vi "exercise8_writetoAO.vi"() -> ()   [LabVIEW 2018]
uses:
  <vilib>/DAQmx/write.llb/DAQmx Write (Analog DBL 1Chan 1Samp).vi
  <vilib>/DAQmx/create/channels.llb/DAQmx Create Channel (AO-Voltage-Basic).vi
  <vilib>/DAQmx/miscellaneous.llb/DAQmx Fill In Error Info.vi
panel:
  out "sampling rate":dbl
  out "error out":errorcluster
  in  "dt (ms)":u32=1
  in  "frequency (Hz)":dbl=1.0
  in  "physical channels":tag="Dev1/ao0"
  out "Waveform Graph":waveform(dbl)(graph)
  out "Waveform Chart":dbl(graph)
  in  "stop":bool
  # "SIGNAL GENERATION: WRITE TO ANALOG OUTPUT"
  # "CHANNEL"
  # "SIGNAL"
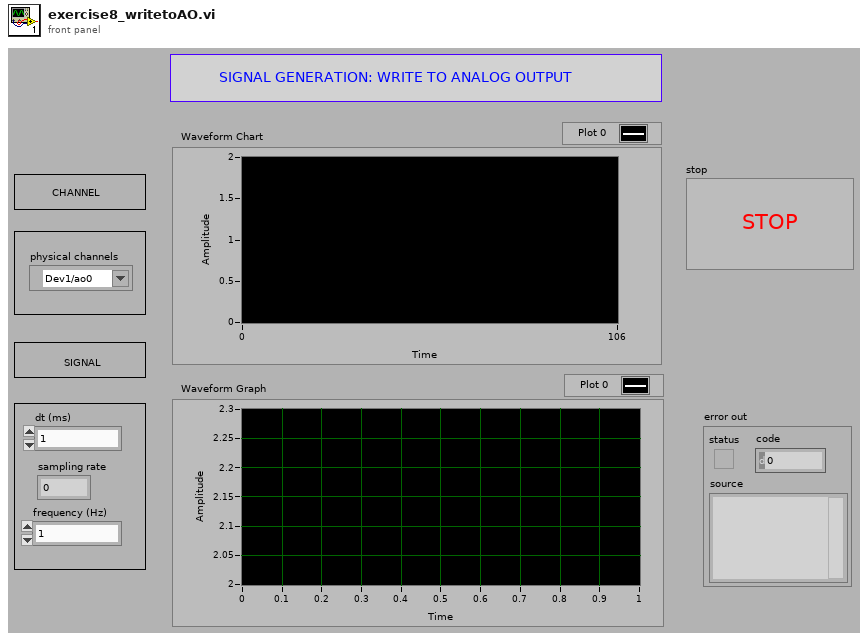
[diagram p1: front panel]
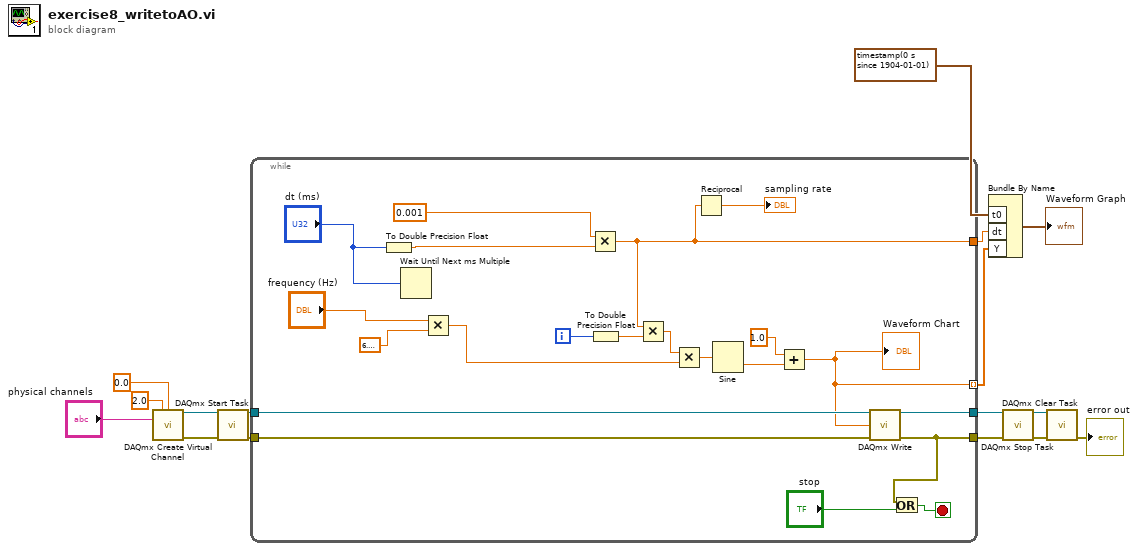
[diagram p0: block diagram]
diagram:
  n1 = call-poly <vilib>:"DAQmx Create Virtual Channel.vi"("maximum value"=2.0, "minimum value"=0.0, "physical channels"="physical channels") -> ("task out"=w9:refnum<k21>, "error out"=w8:errorcluster)  [unwired: 11 in]
  n2 = call <vilib>:"DAQmx Start Task.vi"("task/channels in"=w9, "error in"=w8) -> ("task out"=w16:refnum<k21>, "error out"=w15:errorcluster)  [unwired: 12 in]
  n3 = while {
    tunnel: w16 -> [w36]
    tunnel: w15 -> [w35]
    tunnel: [w37] -> w12
    tunnel: [w25] -> w11
    tunnel: [w33] -> w6 mode=indexing
    tunnel: [w22] -> w1
    i -> [w32]
    stop <- w27 stop-if-true
    n4 = To Double Precision Float(number="dt (ms)") -> (double precision float=w24:dbl)
    n5 = Wait Until Next ms Multiple(millisecond multiple="dt (ms)") -> ()  [unwired: 1 out]
    n6 = Multiply(x="frequency (Hz)", y=6.283185307179586) -> (x*y=w17:dbl)
    n7 = Multiply(x=0.001, y=w24) -> (x*y=w22:dbl)
    n8 = To Double Precision Float(number=w32) -> (double precision float=w30:dbl)
    n9 = Multiply(x=w22, y=w30) -> (x*y=w29:dbl)
    n10 = Multiply(x=w29, y=w17) -> (x*y=w28:dbl)
    n11 = Reciprocal(x=w22) -> (1/x=→"sampling rate":dbl)
    n12 = Sine(x=w28) -> (sin(x)=w34:dbl)
    n13 = Add(x=1.0, y=w34) -> (x+y=w33:dbl)
    "Waveform Chart" <- w33
    n14 = call-poly <vilib>:"DAQmx Write.vi"("task/channels in"=w36, "data"=w33, "error in"=w35) -> ("task out"=w37:refnum<k21>, "error out"=w25:errorcluster)  [unwired: 10 in, 1 out]
    n15 = Or(x=w25, y="stop") -> (x .or. y?=w27:bool)
  }
  n16 = Bundle By Name("t0"=timestamp(0 s since 1904-01-01), "dt"=w1, "Y"=w6) -> (→"Waveform Graph":waveform(dbl))  [unwired: 1 in]
  n17 = call <vilib>:"DAQmx Stop Task.vi"("task/channels in"=w12, "error in"=w11) -> ("task out"=w14:refnum<k21>, "error out"=w13:errorcluster)  [unwired: 12 in]
  n18 = call <vilib>:"DAQmx Clear Task.vi"("task in"=w14, "error in"=w13) -> ("error out"=→"error out":errorcluster)  [unwired: 13 in]
